vi "espectro_hz_base.vi"() -> ()   [LabVIEW 2020]
uses:
  <vilib>/Analysis/NI_AALBase.lvlib
panel:
  in  "Kw":dbl[](array[numeric])
  in  "fs":dbl
  out "FFT":dbl[](graph)
  in  "N FFT":i32=-1
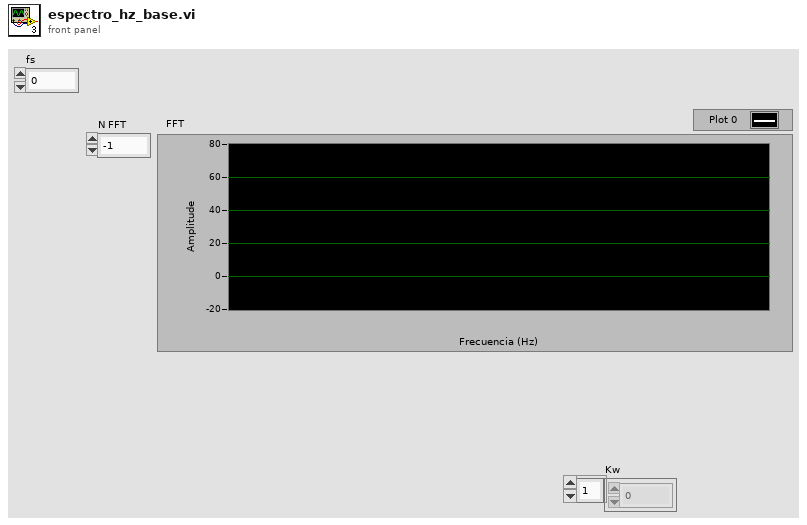
[diagram p1: front panel]
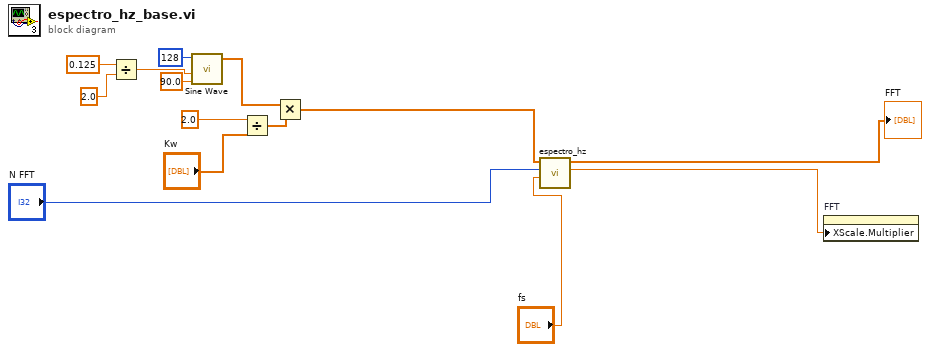
[diagram p0: block diagram]
diagram:
  n1 = Divide(x=0.125, y=2.0) -> (x/y=w9:dbl)
  n2 = call <vilib>:"Sine Wave.vi"("samples"=128, "frequency"=w9, "phase in"=90.0) -> ("sine wave"=w2:dbl[])  [unwired: 2 in, 2 out]
  n3 = Divide(x=2.0, y="Kw") -> (x/y=w5:dbl[])
  n4 = Multiply(x=w2, y=w5) -> (x*y=w1:dbl[])
  n5 = call "espectro_hz.vi"("fs"="fs", "N FFT"="N FFT", "X"=w1) -> ("XScale"=w7:dbl, "FFT(X)"=→"FFT":cdb[])  [unwired: 7 in]
  n6 = property on="FFT" class="WFGraph (strict)"("XScale.Multiplier"=w7) -> ()  [unwired: 2 in, 2 out]
